vi "Row_Combiner.vi"(0 "All Data":string[][](array[string]), 1 "Audit Channels":bool[](array[boolean]), 3 "Coordinates":dbl[](array[numeric]), 5 "Rows to Combine":i32[](array[numeric]), 9 "Position Columns":i32[](array[numeric]), 11 "String In":string, 12 "Include Empty Rows?":bool, 14 "Precision":string[](array[string])) -> (15 "String Out":string)   [LabVIEW 2010]
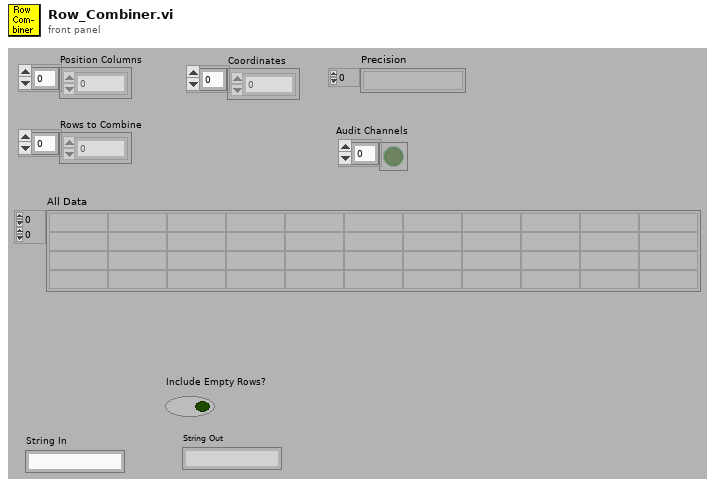
[diagram p1: front panel]
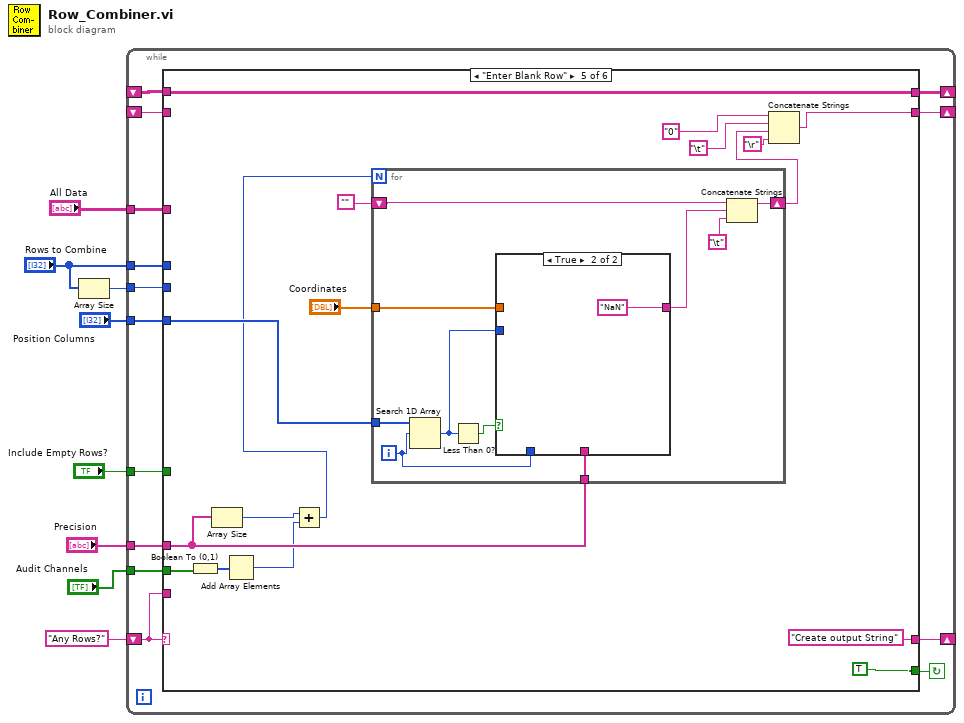
[diagram p0: block diagram]
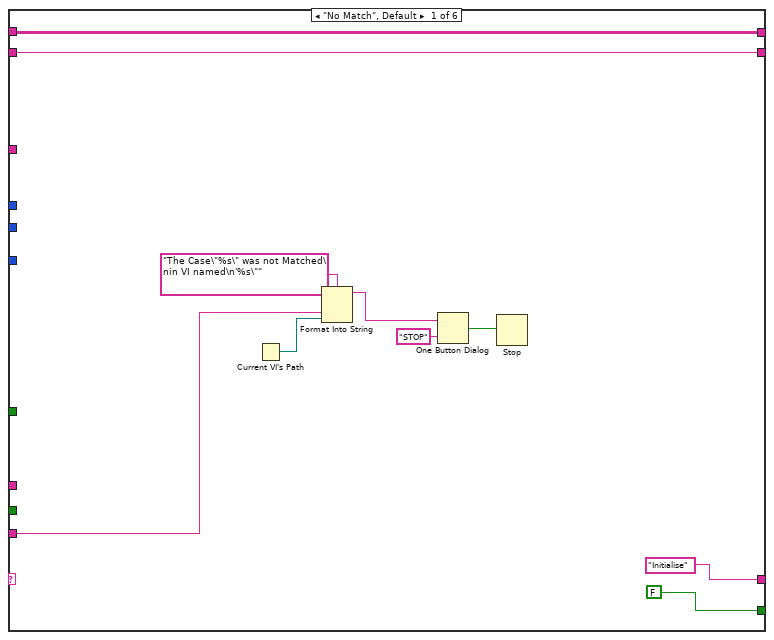
[diagram p2: hidden frame]
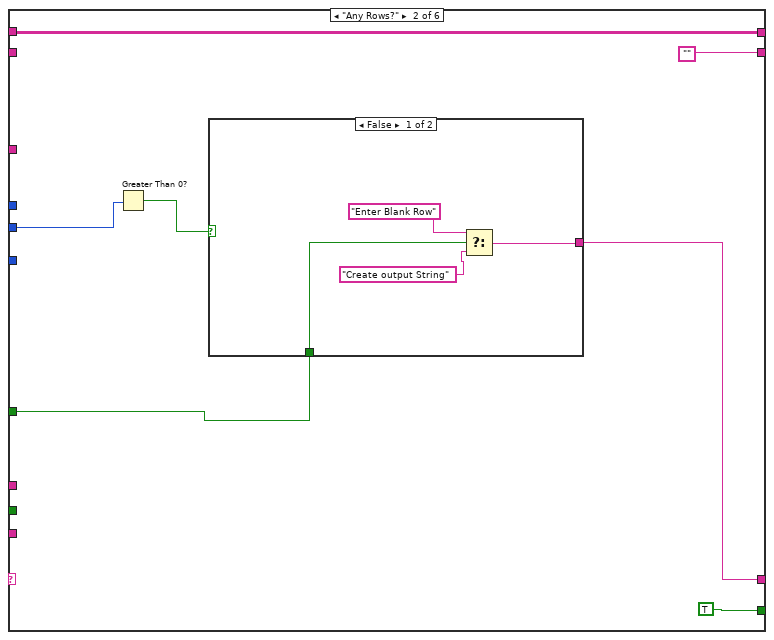
[diagram p3: hidden frame]
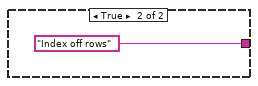
[diagram p4: hidden frame]
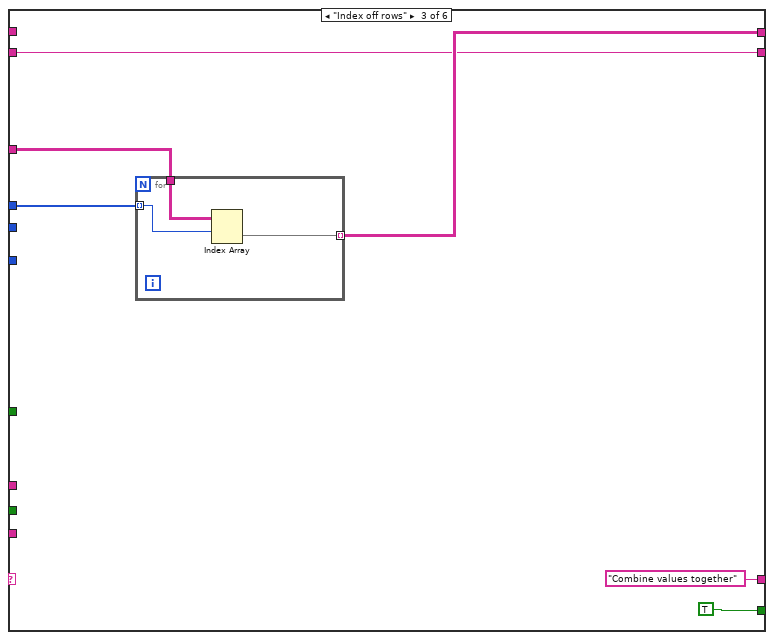
[diagram p5: hidden frame]
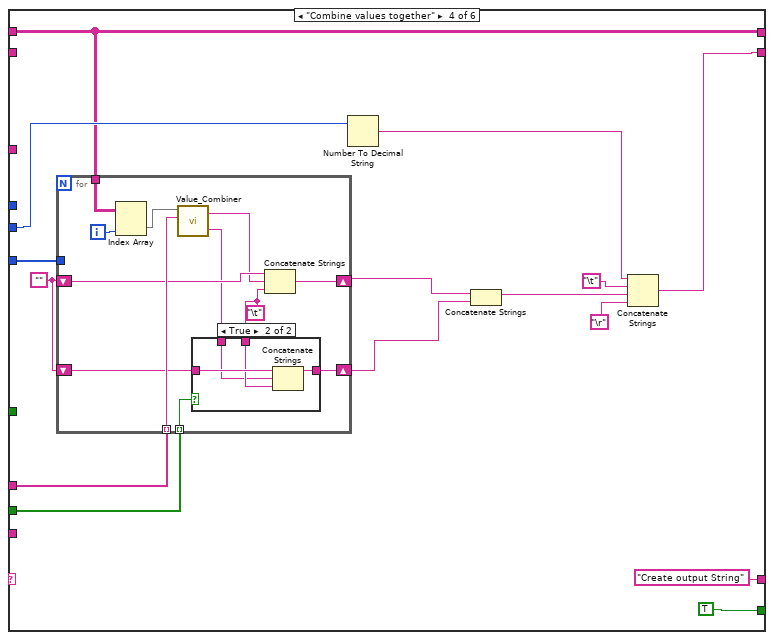
[diagram p6: hidden frame]
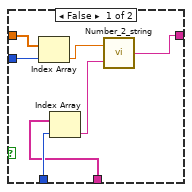
[diagram p8: hidden frame]
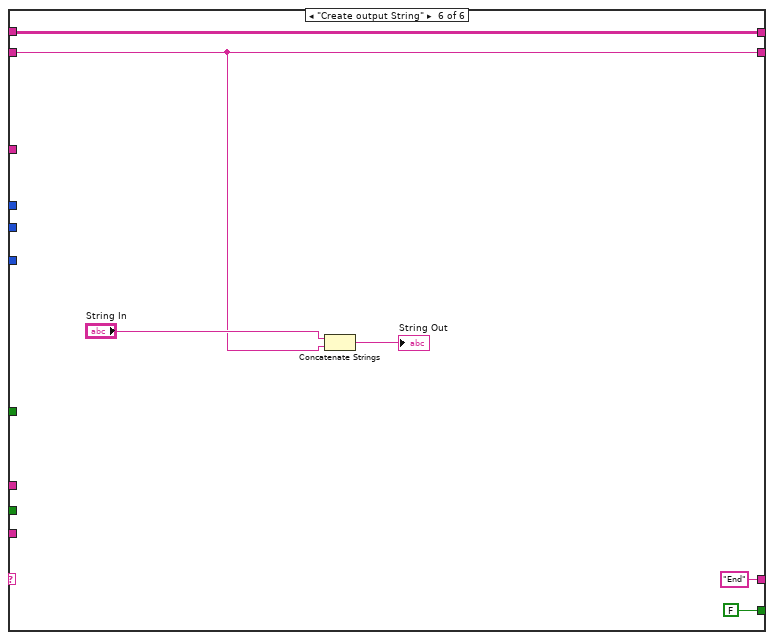
[diagram p9: hidden frame]
diagram:
  n1 = Array Size(array="Rows to Combine") -> (size(s)=w2:i32)
  n2 = while {
    shift-left: "Any Rows?" -> [w20]
    shift-right: [w21] -> _
    shift-right: [w18] -> _
    shift-left: _ -> [w16]
    tunnel: "All Data" -> [w19]
    shift-right: [w17] -> _
    shift-left: _ -> [w15]
    tunnel: "Rows to Combine" -> [w14]
    tunnel: "Include Empty Rows?" -> [w13]
    tunnel: "Position Columns" -> [w12]
    tunnel: "Precision" -> [w11]
    tunnel: w2 -> [w10]
    tunnel: "Audit Channels" -> [w9]
    stop <- w22 continue-if-true
    n3 = case shown="\"Enter Blank Row\"" w20 {
      tunnel: [FALSE TRUE TRUE TRUE TRUE FALSE] -> w22
      tunnel: ["Initialise" w35 "Combine values together" "Create output String" "Create output String" "End"] -> w21
      tunnel: w20 -> [w27 _ _ _ _ _]
      tunnel: w19 -> [_ _ w47 _ _ _]
      tunnel: [w24 w37 w46 w56 w92 w122] -> w18
      tunnel: [w23 "" w45 w60 w94 w121] -> w17
      tunnel: w16 -> [w24 w37 _ w56 w92 w122]
      tunnel: w15 -> [w23 _ w45 _ _ w121]
      tunnel: w14 -> [_ _ w48 _ _ _]
      tunnel: w13 -> [_ w34 _ _ _ _]
      tunnel: w12 -> [_ _ _ w55 w99 _]
      tunnel: w11 -> [_ _ _ w66 w91 _]
      tunnel: w10 -> [_ w33 _ w58 _ _]
      tunnel: w9 -> [_ _ _ w54 w90 _]
      frame "No Match", Default {
        n4 = Current VI's Path() -> (path=w26:path)
        n5 = Format Into String(format string="The Case\"%s\" was not Matched\nin VI named\n'%s\"" ("Format String"), w27, w26) -> (resulting string=w30:string)  [unwired: 2 in, 1 out]
        n6 = One Button Dialog(message=w30, button name ("OK")="STOP") -> (true=w28:bool)
        n7 = Stop(stop? (T)=w28) -> ()
      }
      frame "Any Rows?" {
        n8 = Greater Than 0?(x=w33) -> (x > 0?=w36:bool)
        n9 = case shown="False" w36 {
          tunnel: [w42 "Index off rows"] -> w35
          tunnel: w34 -> [w43 _]
          frame False {
            n10 = Select(t="Enter Blank Row", s=w43, f="Create output String") -> (s? t:f=w42:string)
          }
          frame True {
          }
        }
      }
      frame "Index off rows" {
        n11 = for {
          tunnel: w48 -> [w53] mode=indexing
          tunnel: w47 -> [w52]
          tunnel: [w51] -> w46 mode=indexing
          n12 = Index Array(array=w52, index (row)=w53) -> (element=w51:string[])  [unwired: 1 in]
        }
      }
      frame "Combine values together" {
        w65 = ""
        n13 = for {
          tunnel: w56 -> [w80]
          tunnel: w66 -> [w78] mode=indexing
          shift-right: [w75] -> w64
          shift-left: w65 -> [w77]
          shift-right: [w73] -> w63
          shift-left: w65 -> [w74]
          tunnel: w55 -> [_]
          tunnel: w54 -> [w69] mode=indexing
          i -> [w70]
          w72 = "\t"
          n14 = Index Array(array=w80, index (col)=w70) -> (element=w79:string[])  [unwired: 1 in]
          n15 = call "Value_Combiner.vi"("Precision (3)"=w78, "String Array"=w79) -> ("Audit String"=w71:string, "Output String"=w76:string)  [unwired: 2 out]
          n16 = case shown="True" w69 {
            tunnel: w74 -> [w81 w85]
            tunnel: [w81 w84] -> w73
            tunnel: w72 -> [_ w83]
            tunnel: w71 -> [_ w82]
            frame False {
            }
            frame True {
              n17 = Concatenate Strings(w85, w82, w83) -> (w84:string)
            }
          }
          n18 = Concatenate Strings(w77, w76, w72) -> (w75:string)
        }
        n19 = Number To Decimal String(number=w58) -> (decimal integer string=w57:string)  [unwired: 1 out]
        n20 = Concatenate Strings(w64, w63) -> (w62:string)
        n21 = Concatenate Strings(w57, "\t", w62, "\r") -> (w60:string)
      }
      frame "Enter Blank Row" {
        n22 = Boolean To (0,1)(Boolean=w90) -> (0, 1=w89:i16[])
        n23 = Array Size(array=w91) -> (size(s)=w88:i32)
        n24 = Add Array Elements(numeric array=w89) -> (sum=w87:i16)
        n25 = Add(x=w88, y=w87) -> (x+y=w86:i32)
        n26 = for {
          N: w86 -> [_]
          shift-right: [w111] -> w95
          shift-left: "" -> [w112]
          tunnel: w99 -> [w110]
          tunnel: "Coordinates" -> [w106]
          tunnel: w91 -> [w104]
          i -> [w103]
          n27 = Search 1D Array(1D array=w110, element=w103) -> (index of element=w105:i32)  [unwired: 1 out]
          n28 = Less Than 0?(x=w105) -> (x < 0?=w109:bool)
          n29 = case shown="True" w109 {
            tunnel: [w113 "NaN"] -> w107
            tunnel: w106 -> [w119 _]
            tunnel: w105 -> [w118 _]
            tunnel: w104 -> [w115 _]
            tunnel: w103 -> [w116 _]
            frame False {
              n30 = Index Array(array=w119, index=w118) -> (element=w117:dbl)
              n31 = Index Array(array=w115, index=w116) -> (element=w114:string)
              n32 = call "Number_2_string.vi"("precision"=w114, "number"=w117) -> ("String"=w113:string)
            }
            frame True {
            }
          }
          n33 = Concatenate Strings(w112, w107, "\t") -> (w111:string)
        }
        n34 = Concatenate Strings("0", "\t", w95, "\r") -> (w94:string)
      }
      frame "Create output String" {
        n35 = Concatenate Strings("String In", w121) -> (→"String Out":string)
      }
    }
  }
